vi "Remove Duplicates from 1D.vi"(9 "Input Array":i32[](array[numeric])) -> (1 "No Duplicates Array":i32[](array[numeric]))   [LabVIEW 2016, in "DataGrid.lvlib" / "DataGridView.lvclass"]
doc: "Searches an input array of I32s and outputs the array without any duplicates.\n\n-----\nMike King\nAdvanced Functions Inc.\nOctober 23, 2001"
uses:
  <userlib>/LabVIEWdotNetDataGrid/source/DataGridView/DataGridView.lvclass
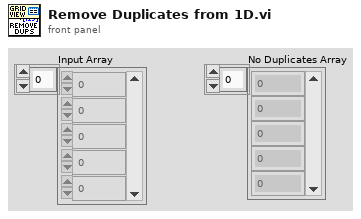
[diagram p1: front panel]
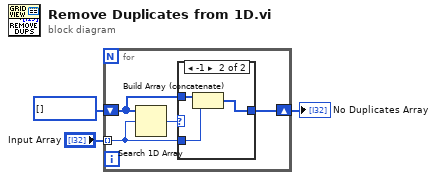
[diagram p0: block diagram]
diagram:
  n1 = for {
    tunnel: "Input Array" -> [w4] mode=indexing
    shift-right: [w5] -> w3
    shift-left: i32[] [] ("Subarray") -> [w6]
    n2 = Search 1D Array(1D array=w6, element=w4) -> (index of element=w7:i32)  [unwired: 1 in]
    n3 = case shown="-1" w7 {
      tunnel: w6 -> [w8 w11]
      tunnel: w4 -> [_ w10]
      tunnel: [w8 w9] -> w5
      frame Default {
      }
      frame -1 {
        n4 = Build Array (concatenate)(w11, w10) -> (w9:i32[])
      }
    }
  }
  "No Duplicates Array" <- w3
